vi "ADIS16448 Scale Data.vi"(8 "error in (no error)":errorcluster, 10 "New Data In":u8[](array[numeric])) -> (0 "error out":errorcluster, 1 "Data Good?":bool, 2 "Data":T1)   [LabVIEW 2019]
panel:
  out "Calculated CRC-16":u16
  out "Received CRC-16":u16
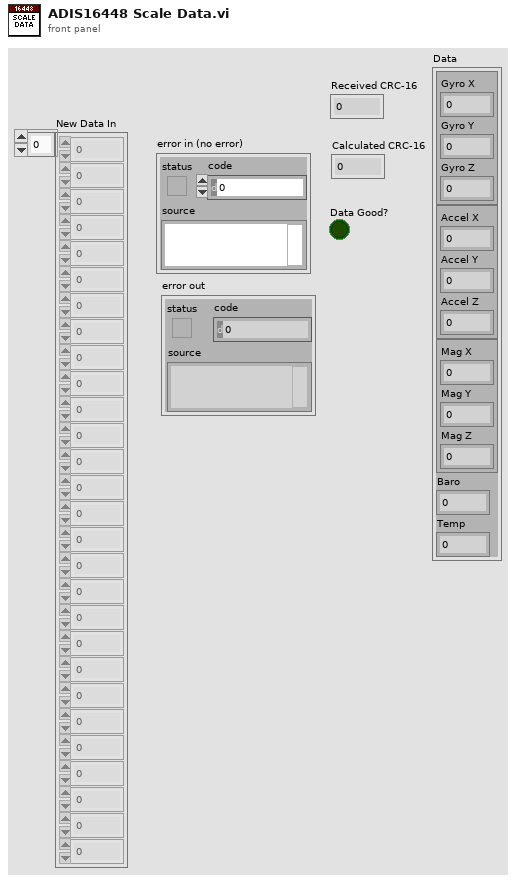
[diagram p1: front panel]
types:
  T1 = cluster{cluster{"Gyro X":dbl, "Gyro Y":dbl, "Gyro Z":dbl}, cluster{"Accel X":dbl, "Accel Y":dbl, "Accel Z":dbl}, cluster{"Mag X":dbl, "Mag Y":dbl, "Mag Z":dbl}, "Baro":dbl, "Temp":dbl}
  T2 = cluster{cluster{"[0]":dbl, "[1]":dbl, "[2]":dbl}, cluster{"[0]":dbl, "[1]":dbl, "[2]":dbl}, cluster{"[0]":dbl, "[1]":dbl, "[2]":dbl}, dbl, dbl}
  T3 = cluster{cluster{"[0]":i16, "[1]":i16, "[2]":i16}, cluster{"[0]":i16, "[1]":i16, "[2]":i16}, cluster{"[0]":i16, "[1]":i16, "[2]":i16}, i16, i16}
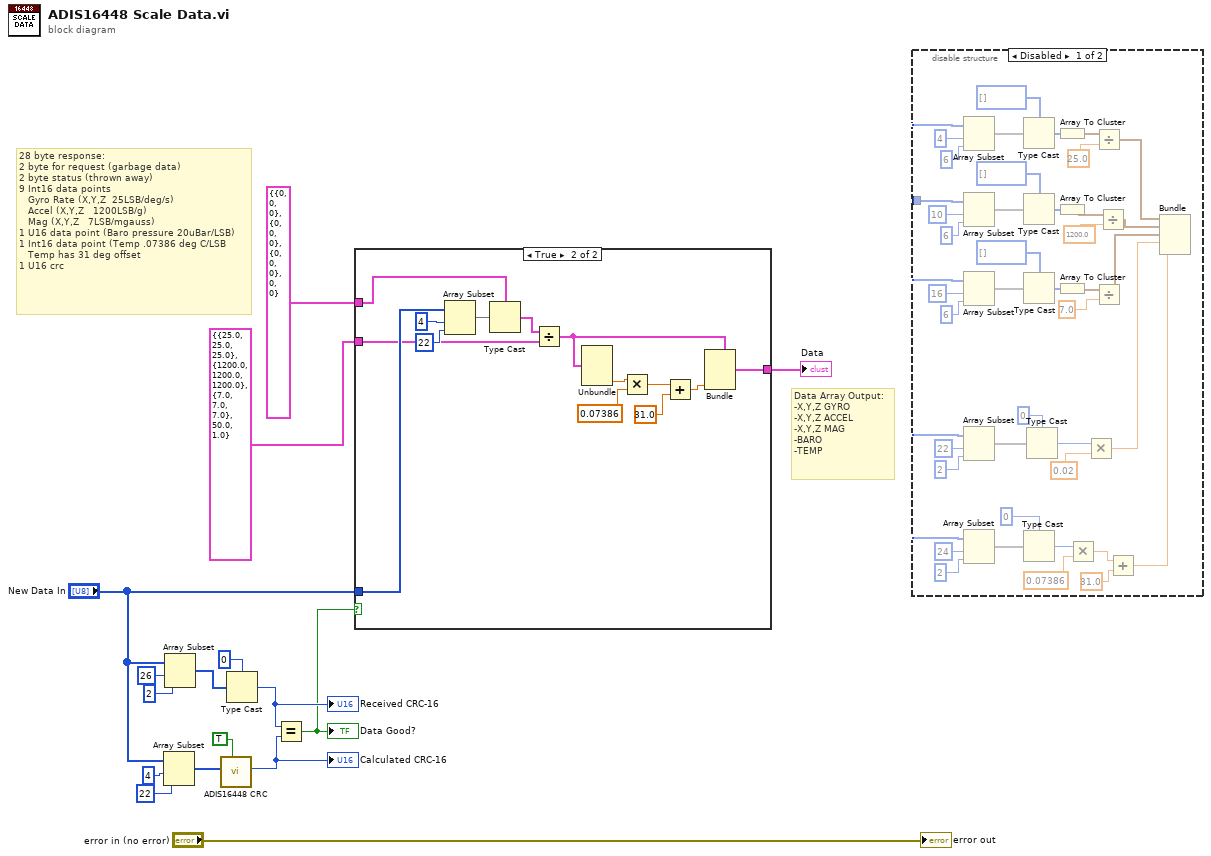
[diagram p0: block diagram]
diagram:
  # "Data Array Output:\n-X,Y,Z GYRO\n-X,Y,Z ACCEL\n-X,Y,Z MAG\n-BARO\n-TEMP"
  # "28 byte response:\n2 byte for request (garbage data)\n2 byte status (thrown away)\n9 Int16 data points\n   Gyro Rate (X,Y,Z  25LSB/deg/s)\n   Accel (X,Y,Z   1200LSB/g)\n   Mag (X,Y,Z   7LSB/mgauss)\n1 U16 data point (Baro pressure 20uBar/LSB)\n1 Int16 data point (Temp .07386 deg C/LSB\n   Temp has 31 deg offset\n1 U16 crc"
  n1 = Array Subset(array="New Data In", index=4, length=22) -> (w8:u8[])
  n2 = Array Subset(array="New Data In", index=26, length=2) -> (w13:u8[])
  n3 = call "ADIS16448 CRC.vi"("Look-Up Table Method?"=TRUE, "Byte Array (MSB-First)"=w8) -> ("CRC16-ADIS"=w7:u16)  [unwired: 9 in]
  "Calculated CRC-16" <- w7
  n4 = Type Cast(type=u16 0, x=w13) -> (*(type *) &x=w10:u16)
  "Received CRC-16" <- w10
  n5 = Equal?(x=w10, y=w7) -> (x = y?=w4:bool)
  "Data Good?" <- w4
  n6 = case shown="True" w4 {
    tunnel: "New Data In" -> [_ w26]
    tunnel: [_ w22] -> w3
    tunnel: T3 {{"[0]"=0, "[1]"=0, "[2]"=0}, {"[0]"=0, "[1]"=0, "[2]"=0}, {"[0]"=0, "[1]"=0, "[2]"=0}, 0, 0} ("Data") -> [_ w30]
    tunnel: T2 {{"[0]"=25.0, "[1]"=25.0, "[2]"=25.0}, {"[0]"=1200.0, "[1]"=1200.0, "[2]"=1200.0}, {"[0]"=7.0, "[1]"=7.0, "[2]"=7.0}, 50.0, 1.0} ("Data") -> [_ w24]
    frame False {
    }
    frame True {
      n7 = Array Subset(array=w26, index=4, length=22) -> (w27:u8[])
      n8 = Type Cast(type=w30, x=w27) -> (*(type *) &x=w25:T3)
      n9 = Divide(x=w25, y=w24) -> (x/y=w23:T2)
      n10 = Unbundle(w23) -> (w19:dbl)  [unwired: 4 out]
      n11 = Multiply(x=w19, y=0.07386 ("element")) -> (x*y=w18:dbl)
      n12 = Add(x=w18, y=31.0) -> (x+y=w17:dbl)
      n13 = Bundle(cluster=w23, w17) -> (w22:T2)  [unwired: 4 in]
    }
  }
  "Data" <- w3
  n14 = disable-structure shown="Disabled" {
    disable-tunnel: _ -> [w31 _]
    frame Disabled {
      n15 = Array Subset(array=w31, index=4, length=6) -> (w55:void[])
      n16 = Array Subset(array=w31, index=10, length=6) -> (w50:void[])
      n17 = Array Subset(array=w31, index=16, length=6) -> (w45:void[])
      n18 = Array Subset(array=w31, index=22, length=2) -> (w61:void[])
      n19 = Array Subset(array=w31, index=24, length=2) -> (w59:void[])
      n20 = Type Cast(type=i16[] [], x=w55) -> (*(type *) &x=w54:i16[])
      n21 = Type Cast(type=i16[] [], x=w50) -> (*(type *) &x=w51:i16[])
      n22 = Type Cast(type=i16[] [], x=w45) -> (*(type *) &x=w44:i16[])
      n23 = Type Cast(type=i16 0, x=w59) -> (*(type *) &x=w56:i16)
      n24 = Type Cast(type=u16 0, x=w61) -> (*(type *) &x=w57:u16)
      n25 = Array To Cluster(array=w54) -> (cluster=w42:cluster{"[0]":i16, "[1]":i16, "[2]":i16})
      n26 = Array To Cluster(array=w51) -> (cluster=w37:cluster{"[0]":i16, "[1]":i16, "[2]":i16})
      n27 = Array To Cluster(array=w44) -> (cluster=w39:cluster{"[0]":i16, "[1]":i16, "[2]":i16})
      n28 = Multiply(x=w56, y=0.07386 ("element")) -> (x*y=w69:dbl)
      n29 = Multiply(x=w57, y=0.02) -> (x*y=w33:dbl)
      n30 = Divide(x=w42, y=25.0 ("element")) -> (x/y=w36:cluster{"[0]":dbl, "[1]":dbl, "[2]":dbl})
      n31 = Divide(x=w39, y=7.0) -> (x/y=w34:cluster{"[0]":dbl, "[1]":dbl, "[2]":dbl})
      n32 = Divide(x=w37, y=1200.0) -> (x/y=w35:cluster{"[0]":dbl, "[1]":dbl, "[2]":dbl})
      n33 = Add(x=w69, y=31.0) -> (x+y=w32:dbl)
      n34 = Bundle(w36, w35, w34, w33, w32) -> ()  [unwired: 1 in, 1 out]
    }
    frame Enabled {
    }
  }
  "error out" <- "error in (no error)"
